vi "ReadDynamixelInformation.vi"(8 "error in (no error)":errorcluster, 9 "Motor ID (0=Main, 1 = Jib)":u8, 10 "VISA resource name":refnum<visa-resource-name>, 11 "Queue in":refnum<queue>) -> (0 "error out":errorcluster)   [LabVIEW 2013]
doc: "Reads Dynamixel torque off of the indicated Dynamixel and writes it to a queue.\n\nEric Schneider, March 2014"
uses:
  <instrlib>/Dynamixel Motor/Dynamixel Motor.lvlib
panel:
  out "Load/torque %":sgl
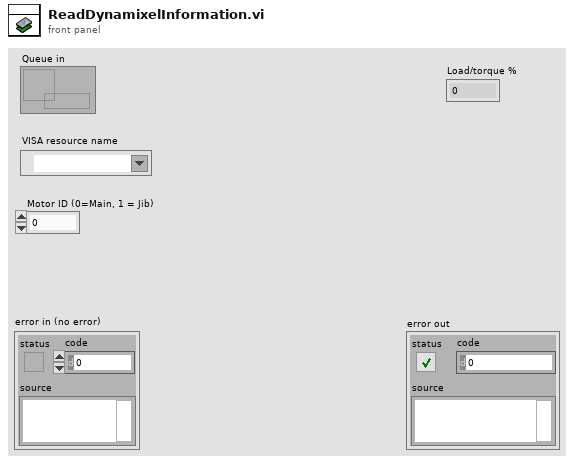
[diagram p1: front panel]
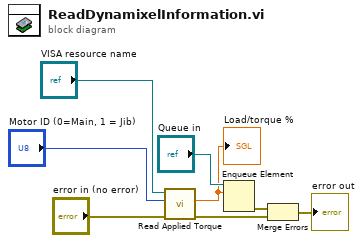
[diagram p0: block diagram]
diagram:
  n1 = call <instrlib>:"Read Applied Torque.vi"("error in (no error)"="error in (no error)", "Motor ID (0)"="Motor ID (0=Main, 1 = Jib)", "VISA resource name"="VISA resource name") -> ("error out"=w3:errorcluster, "Load/torque %"=w4:sgl)  [unwired: 6 in, 1 out]
  "Load/torque %" <- w4
  n2 = Enqueue Element(queue="Queue in", element=w4) -> (error out=w2:errorcluster)  [unwired: 2 in, 2 out]
  n3 = Merge Errors(w2, w3) -> (→"error out":errorcluster)
